vi "TableToWvf(SubVI).vi"(8 "error in":errorcluster, 10 "channel":i32, 11 "ArrayIn":sgl[][](array[numeric])) -> (0 "error IO":errorcluster, 3 "Waveform":waveform(sgl)(graph))   [LabVIEW 2017]
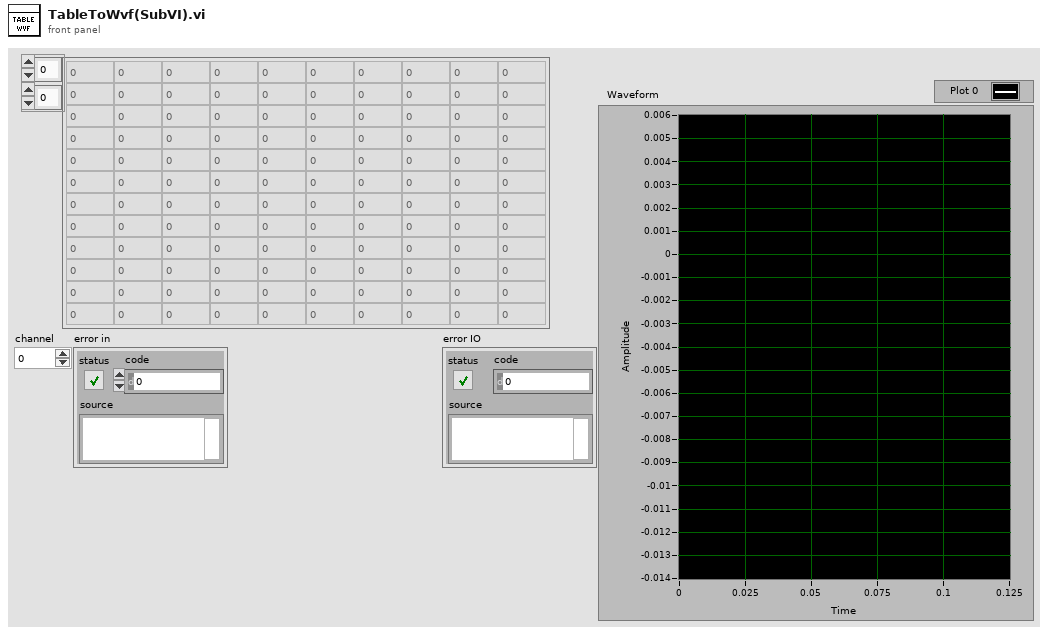
[diagram p1: front panel]
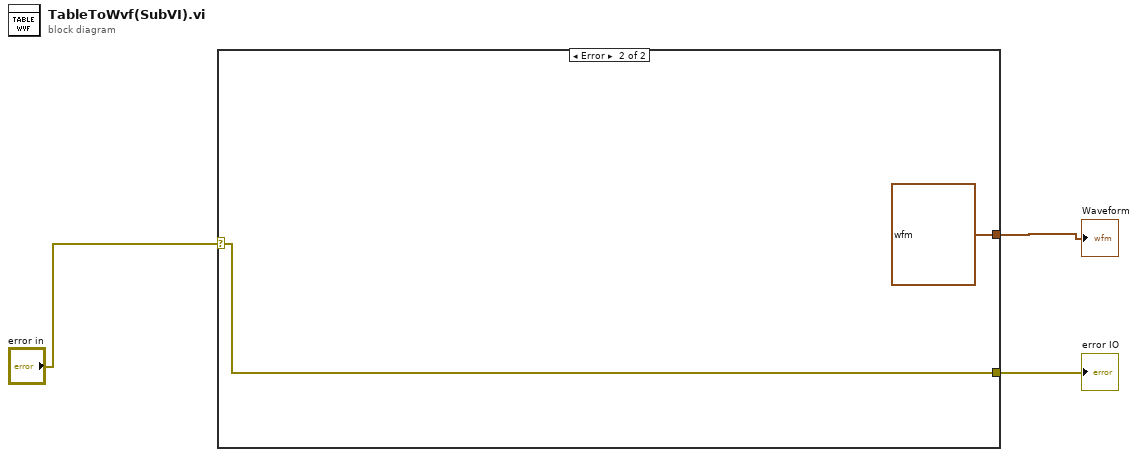
[diagram p0: block diagram]
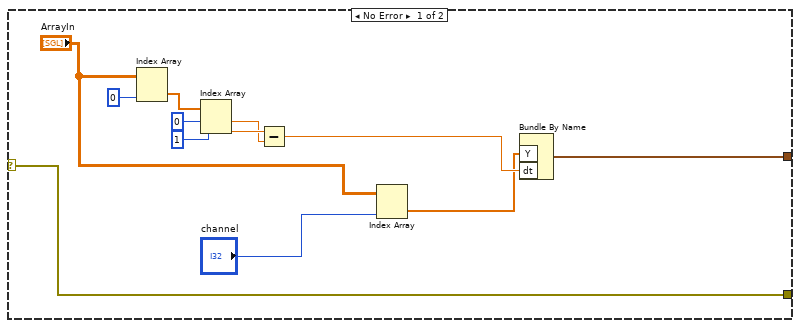
[diagram p2: hidden frame]
diagram:
  n1 = case shown="Error" "error in" {
    selector: "error in" -> [w4 w16]
    tunnel: [w7 waveform(sgl) {"t0"=timestamp(0 s since 1904-01-01), "dt"=1.0, "Y"=[]}] -> w3
    tunnel: [w4 w16] -> w1
    frame No Error {
      n2 = Index Array(array="ArrayIn", index (col)=0 ("disabled index (col)")) -> (element=w13:sgl[])  [unwired: 1 in]
      n3 = Index Array(array=w13, index #1=0 ("index"), index #2=1 ("index")) -> (element #1=w9:sgl, element #2=w10:sgl)
      n4 = Subtract(x=w10, y=w9) -> (x-y=w8:sgl)
      n5 = Index Array(array="ArrayIn", index (col)="channel") -> (element=w6:sgl[])  [unwired: 1 in]
      n6 = Bundle By Name("Y"=w6, "dt"=w8) -> (w7:waveform(sgl))  [unwired: 1 in]
    }
    frame Error {
    }
  }
  "Waveform" <- w3
  "error IO" <- w1
